vi "Floor_Surface_Level.vi"(3 "Simulate/Run":T1, 4 "Traverse Setups":string[](array[string]), 5 "Position In":dbl[](array[numeric])=[0.0, 0.0, 0.0] format="%#.2f") -> (0 "Correct array":bool, 1 "Z Offset":dbl, 2 "Position Out":dbl[](array[numeric]) format="%#.2f")   [LabVIEW 2014]
uses:
  Controls/User_Specific_mode.ctl
  File/Setup_Filetype.ctl
  ADAM Client/Sub VIs/ADAM Controls/Update_scan_value.ctl
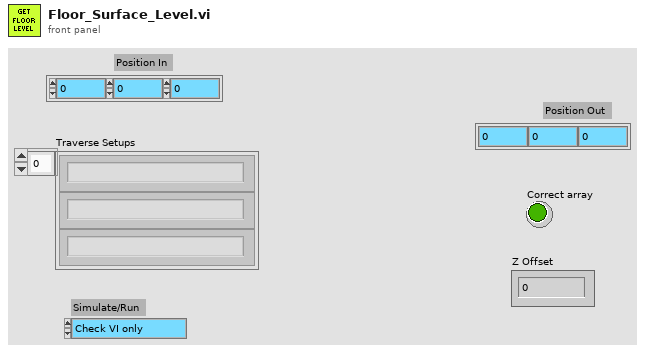
[diagram p1: front panel]
types:
  T1 = typedef "User_Specific_mode.ctl" = enum16{"Check VI only", "Run VI"}
  T2 = typedef "Setup_Filetype.ctl" = enum16{"Measurement Setups", "Calibration Setups", "General", "Results File Plotter Setups", "Speed Calib Tweaks"}
  T3 = typedef "Update_scan_value.ctl" = cluster{"Channel Name":string, "New Value":dbl}
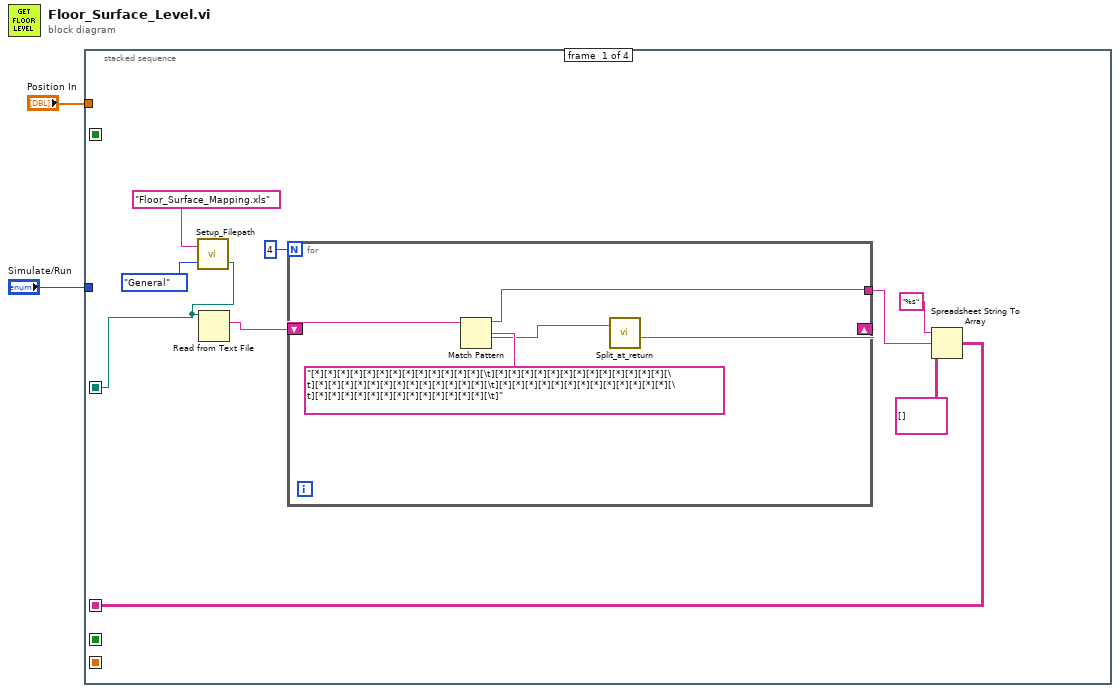
[diagram p0: block diagram]
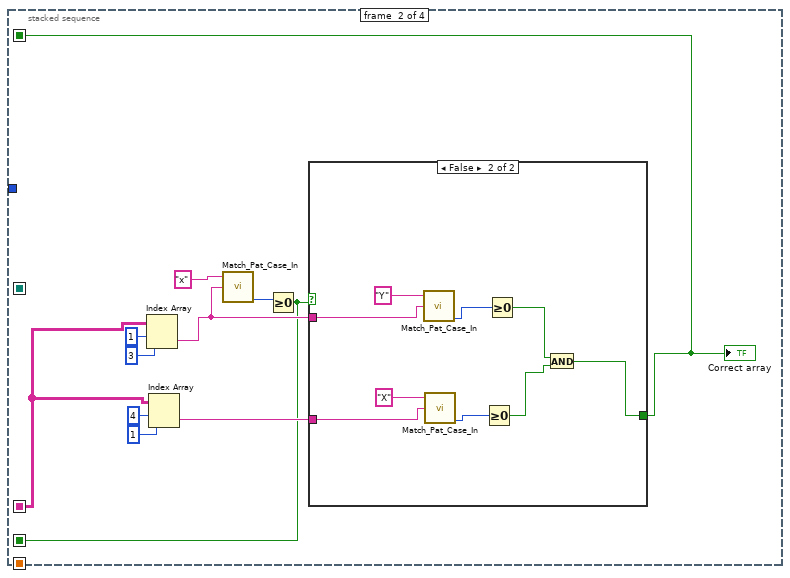
[diagram p2: hidden frame]
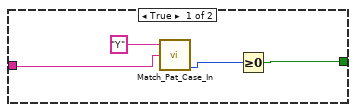
[diagram p3: hidden frame]
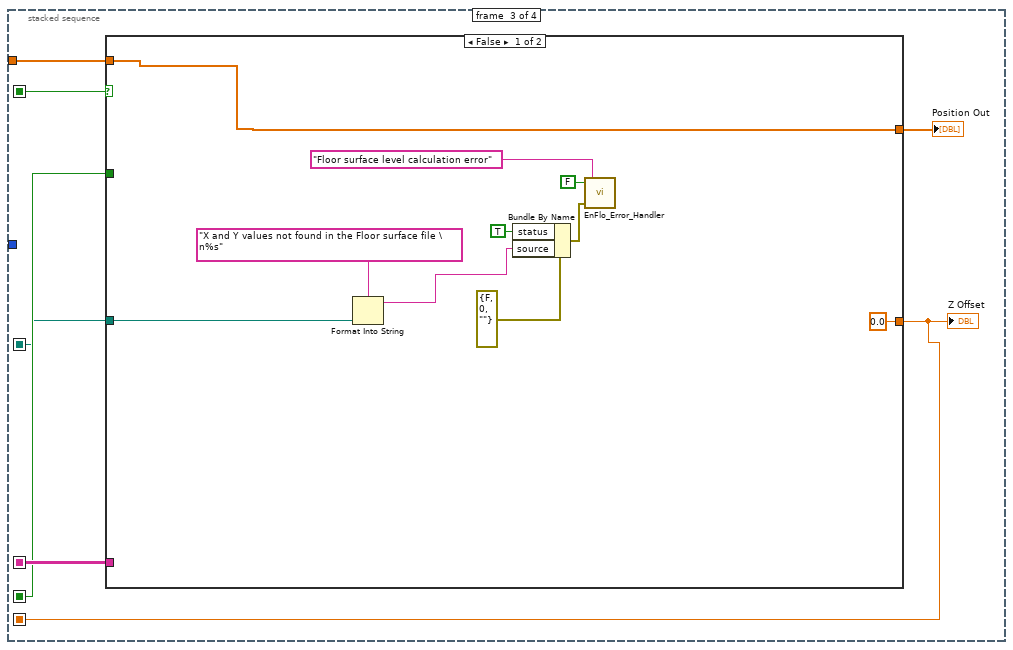
[diagram p4: hidden frame]
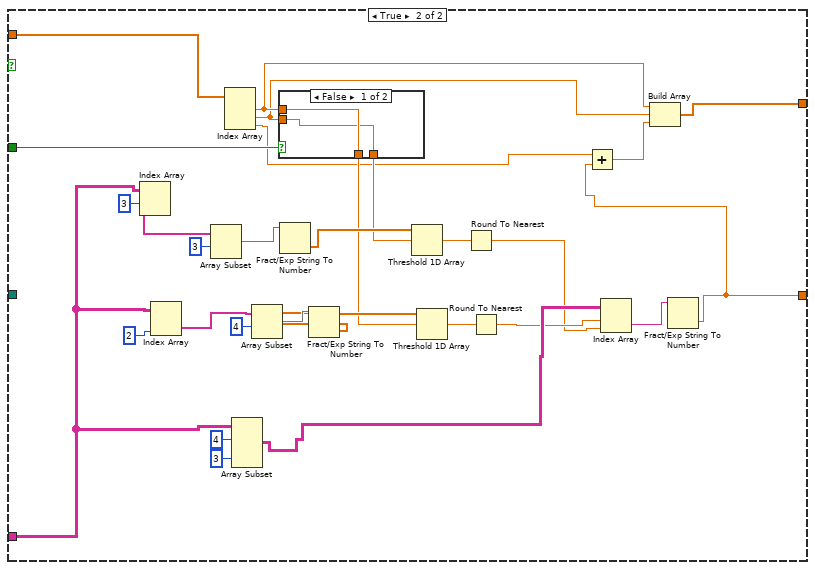
[diagram p5: hidden frame]
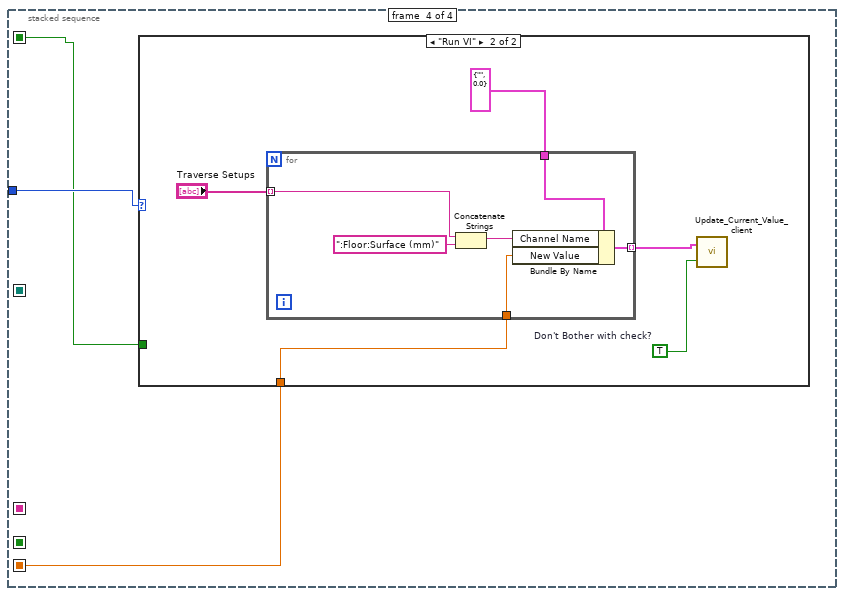
[diagram p7: hidden frame]
diagram:
  n1 = stacked-sequence {
    seq-local: [w6 _ _ _] -> [_ w22 w47 _]
    seq-local: [_ w18 _ _] -> [_ _ w46 _]
    seq-local: [_ _ w42 _] -> [_ _ _ w91]
    seq-local: [_ w17 _ _] -> [_ _ w43 w92]
    seq-local: [w3 _ _ _] -> [_ _ w41 _]
    tunnel: "Simulate/Run" -> [_ _ _ w93]
    tunnel: "Position In" -> [_ _ w44 _]
    frame #0 {
      n2 = call "Setup_Filepath.vi"("Setup File Type"=Setup_Filetype."General", "Filename in"="Floor_Surface_Mapping.xls") -> ("Filename Out"=w3:path)  [unwired: 1 out]
      n3 = Read from Text File(file (use dialog)=w3) -> (text=w11:string)  [unwired: 3 in, 3 out]
      n4 = for {
        N: 4 -> [_]
        shift-right: [w13] -> _
        shift-left: w11 -> [w14]
        tunnel: [w12] -> w8
        n5 = Match Pattern(string=w14, regular expression="[*][*][*][*][*][*][*][*][*][*][*][*][*][\t][*][*][*][*][*][*][*][*][*][*][*][*][*][\t][*][*][*][*][*][*][*][*][*][*][*][*][*][\t][*][*][*][*][*][*][*][*][*][*][*][*][*][\t][*][*][*][*][*][*][*][*][*][*][*][*][*][\t]" ("String")) -> (before substring=w12:string, after substring=w15:string)  [unwired: 3 out]
        n6 = call "Split_at_return.vi"("String"=w15) -> ("after substring"=w13:string)  [unwired: 1 in, 3 out]
      }
      n7 = Spreadsheet String To Array(format string="%s", spreadsheet string=w8, array type (2D Dbl)=string[][] []) -> (array=w6:string[][])  [unwired: 1 in]
    }
    frame #1 {
      n8 = Index Array(array=w22, index (row)=1, index (col)=3) -> (element=w20:string)
      n9 = Index Array(array=w22, index (row)=4, index (col)=1) -> (element=w21:string)
      n10 = call "Match_Pat_Case_In.vi"("String to match"="x", "String"=w20) -> ("offset past match"=w19:i32)  [unwired: 1 in, 3 out]
      n11 = Greater Or Equal To 0?(x=w19) -> (x >= 0?=w18:bool)
      n12 = case shown="False" w18 {
        tunnel: w21 -> [w30 w39]
        tunnel: w20 -> [_ w37]
        tunnel: [w28 w32] -> w17
        frame True {
          n13 = call "Match_Pat_Case_In.vi"("String to match"="Y", "String"=w30) -> ("offset past match"=w29:i32)  [unwired: 1 in, 3 out]
          n14 = Greater Or Equal To 0?(x=w29) -> (x >= 0?=w28:bool)
        }
        frame False {
          n15 = call "Match_Pat_Case_In.vi"("String to match"="Y", "String"=w37) -> ("offset past match"=w36:i32)  [unwired: 1 in, 3 out]
          n16 = call "Match_Pat_Case_In.vi"("String to match"="X", "String"=w39) -> ("offset past match"=w35:i32)  [unwired: 1 in, 3 out]
          n17 = Greater Or Equal To 0?(x=w35) -> (x >= 0?=w34:bool)
          n18 = Greater Or Equal To 0?(x=w36) -> (x >= 0?=w33:bool)
          n19 = And(x=w33, y=w34) -> (x .and. y?=w32:bool)
        }
      }
      "Correct array" <- w17
    }
    frame #2 {
      n20 = case shown="False" w43 {
        tunnel: w47 -> [_ w68]
        tunnel: w46 -> [_ w67]
        tunnel: [0.0 w62] -> w42
        tunnel: [w57 w59] -> w45
        tunnel: w44 -> [w57 w58]
        tunnel: w41 -> [w50 _]
        frame False {
          n21 = Format Into String(format string="X and Y values not found in the Floor surface file \n%s", w50) -> (resulting string=w48:string)  [unwired: 2 in, 1 out]
          n22 = Bundle By Name(cluster=errorcluster {"status"=FALSE, "code"=0, "source"=""} ("error in (no error)"), "status"=TRUE, "source"=w48) -> (w53:errorcluster)
          n23 = call "EnFlo_Error_Handler.vi"("error in (no error)"=w53, "Error Type"="Floor surface level calculation error", "Dialog Box (T)"=FALSE) -> ()  [unwired: 3 out]
        }
        frame True {
          n24 = Index Array(array=w68, index (row)=3) -> (element=w85:string[])  [unwired: 1 in]
          n25 = Index Array(array=w68, index (col)=2 ("index (row)")) -> (element=w81:string[])  [unwired: 1 in]
          n26 = Array Subset(array=w85, index=3) -> (w78:string[])  [unwired: 1 in]
          n27 = Index Array(array=w58) -> (element #1=w64:dbl, element #2=w63:dbl, element #3=w61:dbl)  [unwired: 3 in]
          n28 = Array Subset(array=w68, index (row)=4 ("index"), index (col)=3 ("index")) -> (w72:string[][])  [unwired: 2 in]
          n29 = Array Subset(array=w81, index=4) -> (w77:string[])  [unwired: 1 in]
          n30 = case shown="False" w67 {
            tunnel: w64 -> [w88 w90]
            tunnel: [w87 w90] -> w66
            tunnel: [w88 w89] -> w65
            tunnel: w63 -> [w87 w89]
            frame False {
            }
            frame True {
            }
          }
          n31 = Fract/Exp String To Number(string=w78) -> (number=w76:dbl[])  [unwired: 3 in, 1 out]
          n32 = Fract/Exp String To Number(string=w77) -> (number=w73:dbl[])  [unwired: 3 in, 1 out]
          n33 = Threshold 1D Array(2:w66, 3:w76) -> (0:w75:dbl)  [unwired: 1 in]
          n34 = Threshold 1D Array(2:w65, 3:w73) -> (0:w74:dbl)  [unwired: 1 in]
          n35 = Round To Nearest(number=w75) -> (nearest integer value=w70:dbl)
          n36 = Round To Nearest(number=w74) -> (nearest integer value=w71:dbl)
          n37 = Index Array(array=w72, index (row)=w71, index (col)=w70) -> (element=w69:string)
          n38 = Fract/Exp String To Number(string=w69) -> (number=w62:dbl)  [unwired: 3 in, 1 out]
          n39 = Add(x=w61, y=w62) -> (x+y=w60:dbl)
          n40 = Build Array(w64, w63, w60) -> (w59:dbl[])
        }
      }
      "Z Offset" <- w42
      "Position Out" <- w45
    }
    frame #3 {
      n41 = case shown="\"Run VI\"" w93 {
        tunnel: w92 -> [_ _]
        tunnel: w91 -> [_ w94]
        frame "Check VI only", Default {
        }
        frame "Run VI" {
          w95 = TRUE  # Don't Bother with check?
          n42 = for {
            tunnel: "Traverse Setups" -> [w103] mode=indexing
            tunnel: T3 {"Channel Name"="", "New Value"=0.0} ("Update Scan Value Cluster") -> [w102]
            tunnel: w94 -> [w101]
            tunnel: [w99] -> w96 mode=indexing
            n43 = Concatenate Strings(w103, ":Floor:Surface (mm)" ("string")) -> (w100:string)
            n44 = Bundle By Name(cluster=w102, "Channel Name"=w100, "New Value"=w101) -> (w99:T3)
          }
          n45 = call "Update_Current_Value_client.vi"("Don't Bother with check?"=w95, "Update array in"=w96) -> ()
        }
      }
    }
  }
